vi "VCA_M.vi"(4 "Amount?":bool, 6 "EG":fxp<+,8,0>=0.99609375, 7 "Scale":i8, 9 "LFO":fxp<+/-,8,8>, 10 "Amount":fxp<+,8,0>, 11 "Sample In":fxp<+/-,8,8>) -> (3 "Sample Out":fxp<+/-,8,8>)   [LabVIEW 2015]
doc: "Performs static and dynamic amplitude control, and allows disabling of the input 'Amount', for example for minimum attenuation at the start of a sound.\n\nThe latency of this VI is 21 cycles."
uses:
  <vilib>/rvi/FXPMathLib/FxpMul/XNode/nifxpmath_Multiplier.xnode
  <vilib>/rvi/FXPMathLib/sim/FxpSim.dll
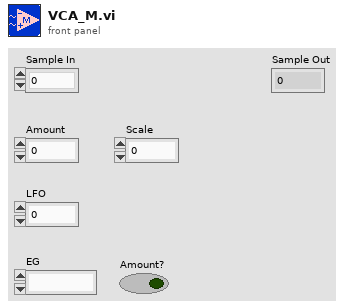
[diagram p1: front panel]
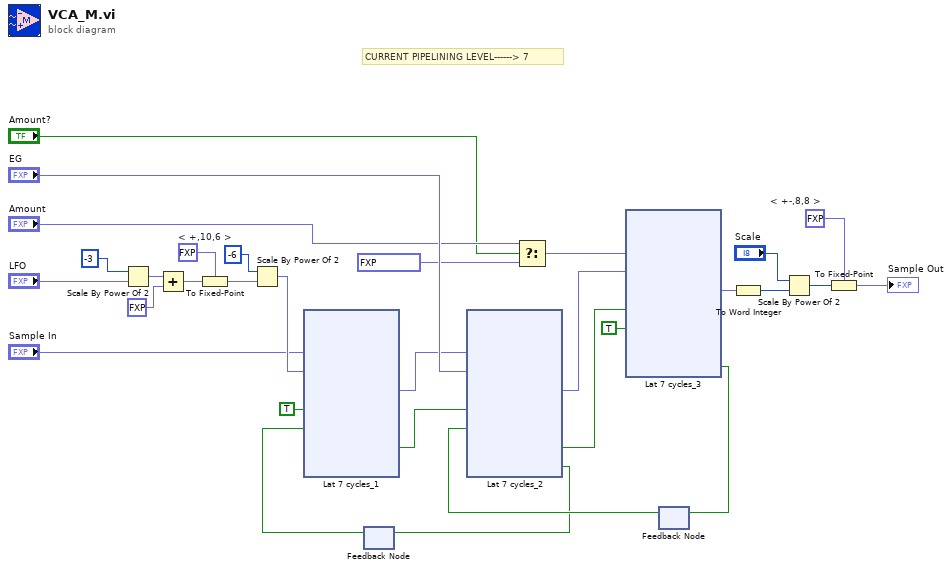
[diagram p0: block diagram]
diagram:
  w1 = fxp<+/-,8,8> 0.0  # < +-,8,8 >
  w24 = fxp<+,10,6> 0.0  # < +,10,6 >
  # "CURRENT PIPELINING LEVEL------> 7"
  n1 = Scale By Power Of 2(n=i8 -3, x="LFO") -> (x*2^n=w27:fxp<+/-,8,8>)
  n2 = Add(x=w27, y=fxp<+/-,8,8> 48.0 ("Amount")) -> (x+y=w25:fxp<+/-,9,9>)
  n3 = To Fixed-Point(fixed-point type=w24, number=w25) -> (fixed-point=w23:fxp<+,10,6>)
  n4 = Scale By Power Of 2(n=i8 -6, x=w23) -> (x*2^n=w21:fxp<+,10,6>)
  n5 = feedback #1() -> (w10:bool)  [unwired: 1 in]
  n6 = xnode "Lat 7 cycles_1"("x"="Sample In", "y"=w21, "input valid"=TRUE, "ready for output (T)"=w10) -> ("x*y"=w30:fxp<+/-,18,14>, "output valid"=w9:bool)  [unwired: 1 out]
  n7 = Select(t="Amount", s="Amount?", f=fxp<+,8,0> 0.99609375 ("s? t:f")) -> (s? t:f=w6:fxp<+,8,0>)
  n8 = feedback #2() -> (w13:bool)  [unwired: 1 in]
  n9 = xnode "Lat 7 cycles_2"("x"=w30, "y"="EG", "input valid"=w9, "ready for output (T)"=w13) -> ("x*y"=w20:fxp<+/-,26,14>, "output valid"=w8:bool, "ready for input"=w11:bool)
  n10 = feedback-in #1(w11) -> ()
  n11 = xnode "Lat 7 cycles_3"("x"=w6, "y"=w20, "input valid"=w8, "ready for output (T)"=TRUE) -> ("x*y"=w18:fxp<+/-,34,14>, "ready for input"=w14:bool)  [unwired: 1 out]
  n12 = feedback-in #2(w14) -> ()
  n13 = To Word Integer(number=w18) -> (16bit integer=w17:i16)
  n14 = Scale By Power Of 2(n="Scale", x=w17) -> (x*2^n=w16:i16)
  n15 = To Fixed-Point(fixed-point type=w1, number=w16) -> (fixed-point=→"Sample Out":fxp<+/-,8,8>)
